vi "Override Config File Path.vi"(8 "error in (no error)":errorcluster, 10 "Config File Path":path, 11 "Output Actor Hardware Interface in":refnum<class "Output Actor Hardware Interface.lvclass">) -> (0 "error out":errorcluster, 3 "Output Actor Hardware Interface out":refnum<class "Output Actor Hardware Interface.lvclass">)   [LabVIEW 2015, in "Output Actor Hardware Interface.lvclass"]
uses:
  Output Actor Hardware Interface.lvclass
  Output Actor Hardware Interface.lvclass/Output Actor Hardware Interface.ctl
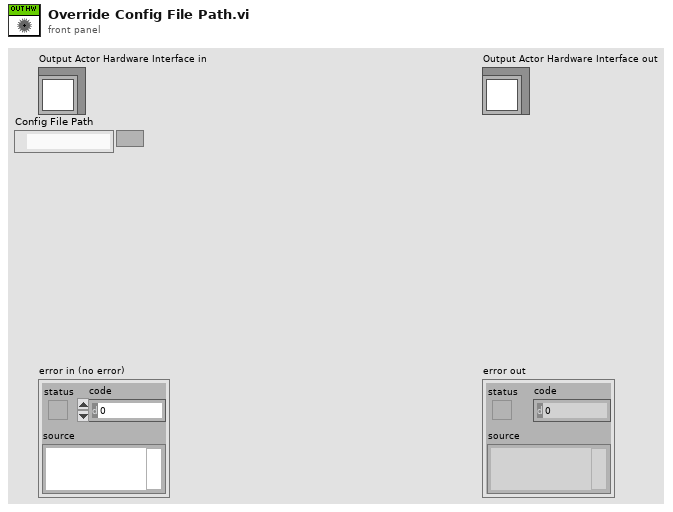
[diagram p1: front panel]
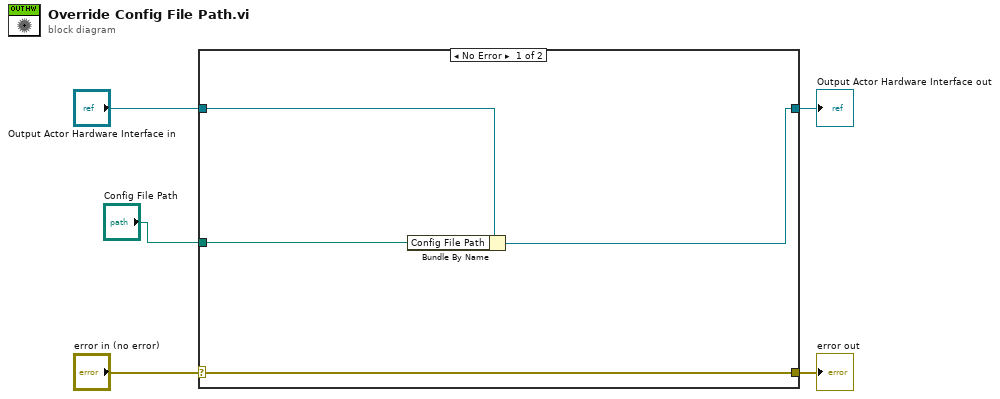
[diagram p0: block diagram]
diagram:
  n1 = case shown="No Error" "error in (no error)" {
    selector: "error in (no error)" -> [w9 w11]
    tunnel: [w9 w11] -> w4
    tunnel: [w8 w10] -> w2
    tunnel: "Output Actor Hardware Interface in" -> [w7 w10]
    tunnel: "Config File Path" -> [w6 _]
    frame No Error {
      n2 = Bundle By Name(cluster=w7, "Config File Path"=w6) -> (w8:refnum<class "Output Actor Hardware Interface.lvclass">)
    }
    frame Error {
    }
  }
  "error out" <- w4
  "Output Actor Hardware Interface out" <- w2
